vi "SelectMenuRuntime.vi"(0 "XRef":T7, 1 "Item Index":T6, 2 "Id":T5, 3 "Point":T3, 4 "State In":T2) -> (14 "Fatal Error Out":T1)   [LabVIEW 2022 SP3, in "Flex Block.xnode"]
uses:
  Flex Block.xnode
  <vilib>/XNodeSupport/XNodeXNodeRef.ctl
  <vilib>/XNodeSupport/XNodeUInt.ctl
  <vilib>/XNodeSupport/XNodeString.ctl
  <vilib>/XNodeSupport/XNodePoint.ctl
  <vilib>/XNodeSupport/XNodeInt.ctl
  State.ctl
  <vilib>/XNodeSupport/XNodeErrorCluster.ctl
  <vilib>/XNodeSupport/NI_XNodeSupport.lvlib
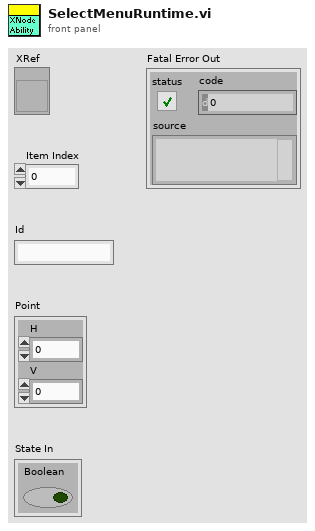
[diagram p1: front panel]
types:
  T1 = typedef "NI_XNodeSupport.lvlib/XNodeErrorCluster.ctl" = errorcluster
  T2 = typedef "Flex Block.xnode/State.ctl" = cluster{"Boolean":bool}
  T3 = typedef "NI_XNodeSupport.lvlib/XNodePoint.ctl" = cluster{"H":T4, "V":T4}
  T4 = typedef "NI_XNodeSupport.lvlib/XNodeInt.ctl" = i32
  T5 = typedef "NI_XNodeSupport.lvlib/XNodeString.ctl" = string
  T6 = typedef "NI_XNodeSupport.lvlib/XNodeUInt.ctl" = u32
  T7 = typedef "NI_XNodeSupport.lvlib/XNodeXNodeRef.ctl" = refnum<vi>
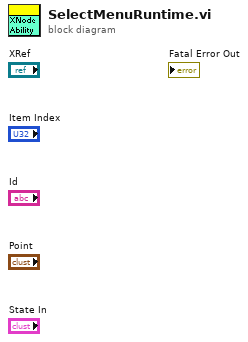
[diagram p0: block diagram]
diagram:
